vi "DSF.Engine.Framework.Get Engine Pointer.vi"(11 "Framework in":refnum<class "DSF.Engine.Framework.lvclass">) -> (2 "Engine Pointer":refnum<class "Memory.Pointer.lvclass">, 3 "Framework out":refnum<class "DSF.Engine.Framework.lvclass">)   [LabVIEW 2017, in "DSF.Engine.lvlib" / "DSF.Engine.Framework.lvclass"]
uses:
  DSF.Engine.Framework.lvclass
  <vilib>/National Instruments/Memory Manager/Classes/Pointer/Memory.Pointer.lvclass
  DSF.Engine.Framework.lvclass/DSF.Engine.Framework.ctl
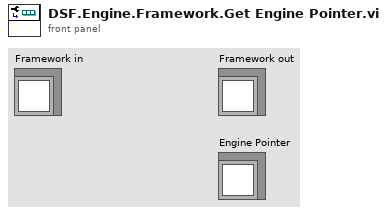
[diagram p1: front panel]
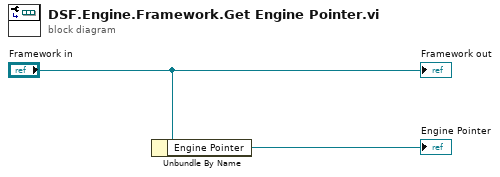
[diagram p0: block diagram]
diagram:
  n1 = Unbundle By Name("Framework in") -> ("Engine Pointer"=→"Engine Pointer":refnum<class "Memory.Pointer.lvclass">)
  "Framework out" <- "Framework in"
